vi "ExTestColi32.vi"() -> ()   [LabVIEW 2010]
panel:
  in  "Column":u32=1 min=1
  in  "Row":u32=1 min=1
  out "Row":i32[](graph)
  out "Column":i32[](graph)
  out "error out":errorcluster
  in  "error in (no error)":errorcluster
  out "Image Display":i32[][](graph)
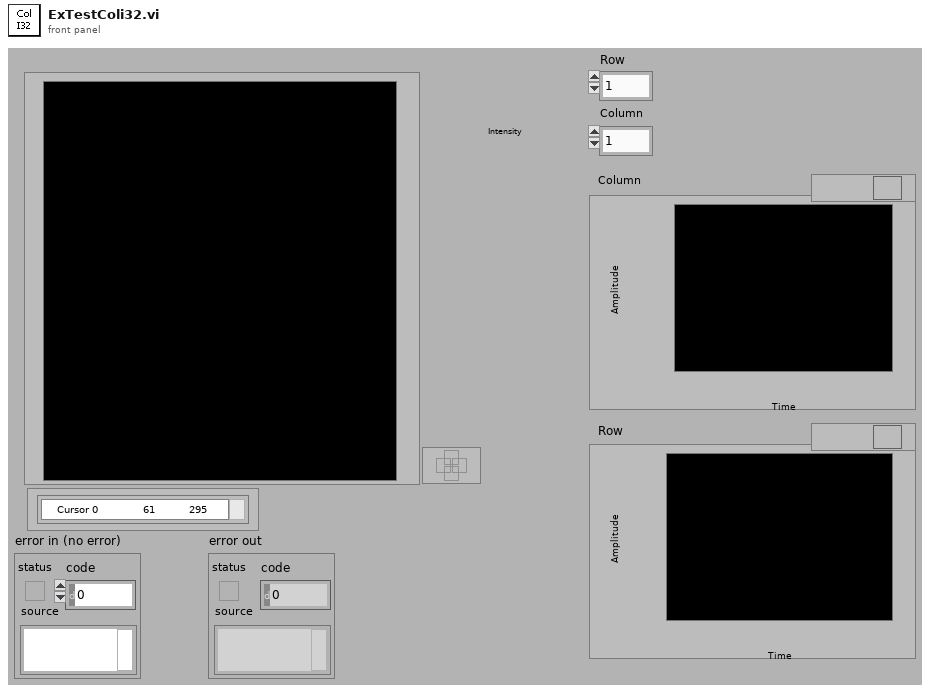
[diagram p1: front panel]
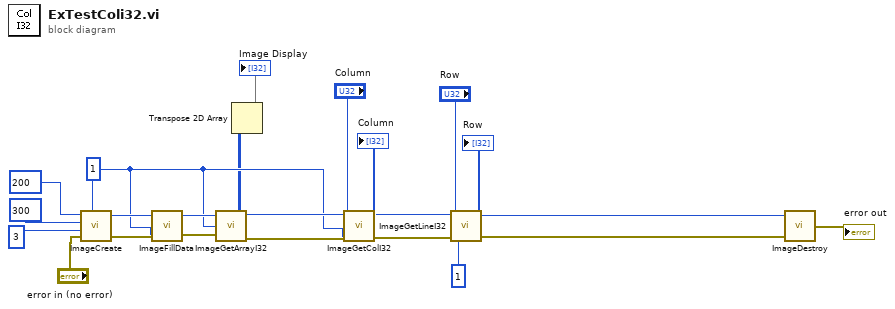
[diagram p0: block diagram]
diagram:
  w12 = 1
  n1 = call <userlib>:"ImageCreate.vi"("X dimension"=200, "Y dimension"=300, "Data Type"=3, "error in"="error in (no error)", "Number Of Frames"=w12) -> ("Image Handle"=w18:u32, "error out"=w19:errorcluster)
  n2 = call <userlib>:"ImageFillData.vi"("error in"=w19, "Type of Test"=w12, "Image Handle"=w18) -> ("error out"=w17:errorcluster, "Image Handle"=w16:u32)
  n3 = call <userlib>:"ImageGetArrayI32.vi"("error in"=w17, "Z position"=w12, "Image Handle"=w16) -> ("error out"=w14:errorcluster, "Array int 32"=w10:i32[][], "Image Handle"=w13:u32)
  n4 = Transpose 2D Array(2D array=w10) -> (transposed array=→"Image Display":i32[][])
  n5 = call <userlib>:"ImageGetColI32.vi"("error in (no error)"=w14, "Z position"=w12, "X position"="Column", "Image Handle"=w13) -> ("error out"=w7:errorcluster, "Array I32"=→"Column":i32[], "Image Handle"=w6:u32)
  n6 = call <userlib>:"ImageGetLineI32.vi"("error in"=w7, "Z Position"=1, "Y Position"="Row", "Data Handle"=w6) -> ("error out"=w3:errorcluster, "Array i32"=→"Row":i32[], "Data Handle"=w2:u32)
  n7 = call <userlib>:"ImageDestroy.vi"("error in"=w3, "Data handle"=w2) -> ("error out"=→"error out":errorcluster)
